vi "Evaluate 3D Polynomial.vi"(7 "Highest order":i32=1, 8 "error in":errorcluster, 9 "Coefficients":dbl[](array[numeric]) format="%.3e", 10 "Y":dbl[](array[numeric]), 11 "X":dbl[](array[numeric])) -> (0 "error out":errorcluster, 2 "Z":dbl[](array[numeric]) format="%.2f")   [LabVIEW 2009]
doc: "This .vi returns the Z points for the input X,Y coordinates and polynomial coefficients. The coeffs are generated from the 3d poly fit."
uses:
  <vilib>/Analysis/baseanly.llb/A x Vector.vi
  <vilib>/Analysis/NI_AALBase.lvlib
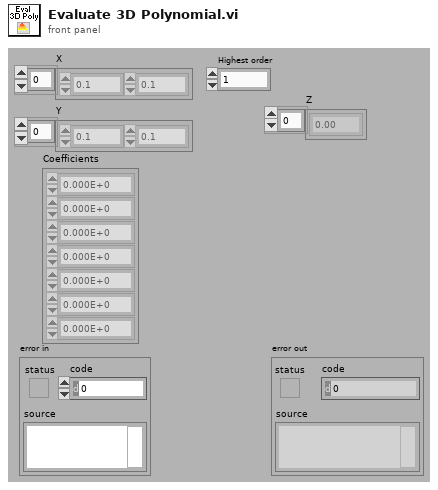
[diagram p1: front panel]
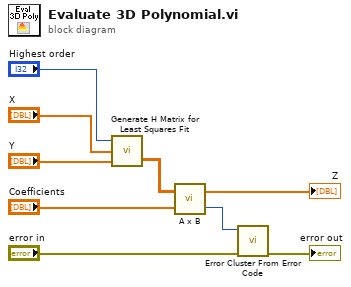
[diagram p0: block diagram]
diagram:
  n1 = call "Generate H Matrix for Least Squares Fit.vi"("[Y]"="Y", "[X]"="X", "Highest order"="Highest order") -> ("H"=w9:dbl[][])  [unwired: 1 out]
  n2 = call-poly <vilib>:"A x B.vi"("Vector"="Coefficients", "A"=w9) -> ("error"=w3:i32, "A x Vector"=→"Z":dbl[])
  n3 = call <vilib>:"Error Cluster From Error Code.vi"("error in (no error)"="error in", "error code (0)"=w3) -> ("error out"=→"error out":errorcluster)  [unwired: 1 in, 6 out]
